vi "Main.vi"() -> ()   [LabVIEW 2016]
uses:
  <vilib>/Platform/TimedLoop/XDataNode/timing_clust.ctl
  <vilib>/Platform/TimedLoop/XDataNode/nitl_modes.ctl
  <vilib>/Platform/TimedLoop/XDataNode/wakeup.ctl
  <vilib>/rvi/Emulation/niFpgaGetClockAttributes.vi
  <vilib>/rvi/Emulation/niFpgaSctlEmulationGetInTimedLoop.vi
  <vilib>/rvi/Emulation/niFpgaEmulationReportErrorSimple.vi
  <vilib>/rvi/Emulation/niFpgaCriticalErrorInLSC.vi
  <vilib>/rvi/Emulation/niFpgaEmulationIsFPGAContextNoSignature.vi
  <vilib>/rvi/DataTransferAndStorage/Container/Common/niFpgaContainerGetUniqueNameForEmu.vi
  <vilib>/rvi/Memory/Memory_Emulation/niFpgaMemoryEmulationCacheClearOnFirstRun.vi
  <vilib>/rvi/Memory/Memory_Emulation/nirvimemoryEmulationManagerCache_MakeExclusive.vi
  <vilib>/rvi/Memory/Memory_Emulation/niFpgaMemoryEmulationValidateCache.vi
  <vilib>/rvi/Memory/Memory_Emulation/nirvimemoryEmulationManagerCache_InsertValue.vi
  <vilib>/Utility/error.llb/Clear Errors.vi
  <vilib>/rvi/Memory/Memory_Emulation/nirvimemoryEmulationManagerCache_ReleaseExclusive.vi
  <vilib>/rvi/Memory/Memory_Emulation/nirvimemoryEmulationManagerCache_GetValue.vi
  <vilib>/rvi/Memory/Memory_Emulation/nirvimemoryEmulationManagerCache_SetValue.vi
  <vilib>/rvi/Emulation/niFpgaProcessEmulError.vi
  <vilib>/rvi/Memory/Memory_Emulation/nirvimemoryFastEmulation.vi
  <vilib>/rvi/Memory/Memory_Emulation/nirvimemoryEmulation.vi
  <vilib>/rvi/errors/nirviReportUnexpectedCaseInternalError (U32).vi
  <vilib>/rvi/DataTransferAndStorage/Container/Common/niFpgaContainerExecOnDevCompGetState.vi
  <vilib>/rvi/Emulation/niFpgaSctlEmulationResourceMgr.vi
  <vilib>/Platform/TimedLoop/XDataNode/XDataNode.xnode
  <vilib>/rvi/DataTransferAndStorage/Container/XNode/niFpgaContainer.xnode
  <vilib>/rvi/DataTransferAndStorage/Register/Emulation/niFpgaRegisterEmulation.vi
  <vilib>/rvi/Memory/Memory_Emulation/niFpgaMemoryEmulationRefIn.vi
  <vilib>/Platform/TimedLoop/XDataNode/XDNodeRunTimeDep.lvlib
panel:
  out "Flags":u8
  out "InclinometerAngle":u32
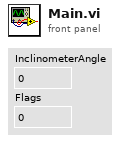
[diagram p1: front panel]
types:
  T1 = typedef "XDNodeRunTimeDep.lvlib/timing_clust.ctl" = cluster{"Expected End [f-1]":u64, "Actual End [f-1]":u64, "Finished Late? [f-1]":bool, "Expected End [i-1]":u64, "Actual End [i-1]":u64, "Finished Late? [i-1]":bool, "Expected Start [i]":u64, "Actual Start [i]":u64, "Expected Start [f]":u64, "Actual Start [f]":u64, "Source Name":string, "Structure Name":string, "Period":i64, "Deadline":i64, "Offset":i64, "Start":i64, "Priority":i32, "Timeout":i32, "Mode":T2, "Wakeup Reason":T3, "Error":errorcluster, "Source Type":string, "Secondary Source Type":string, "Global End Time":u64, "Global Start Time":u64, "Frame Duration":u64, "Iteration Duration":u64, "Assigned CPU":i32, "I/O Scan Engine Mode":u32}
  T2 = typedef "XDNodeRunTimeDep.lvlib/nitl_modes.ctl" = enum32{"No Change", "Process missed periods, maintain original phase", "Discard missed periods, maintain original phase", "Process missed periods, ignore original phase", "Discard missed periods, ignore original phase"}
  T3 = typedef "XDNodeRunTimeDep.lvlib/wakeup.ctl" = enum32{"Normal", "Aborted", "Asynchronous wakeup", "Timing source error", "Timed loop error", "Timeout"}
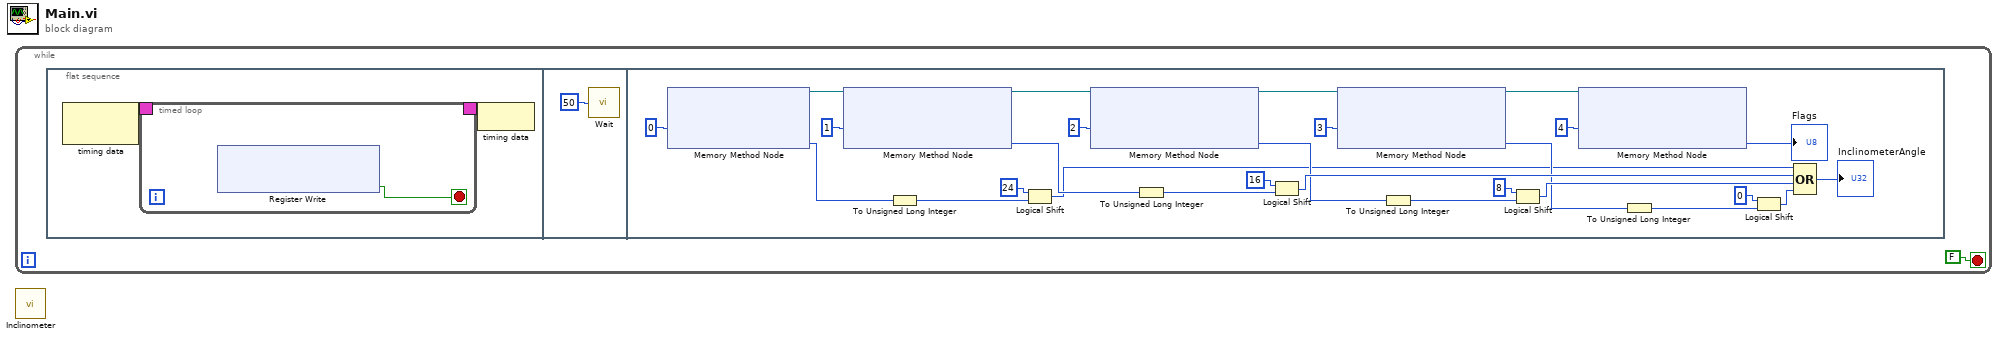
[diagram p0: block diagram]
diagram:
  n1 = while {
    stop <- FALSE stop-if-true
    n2 = flat-sequence {
      frame #0 {
        n3 = node-c288() -> (w3:T1)  [unwired: 1 in]
        n4 = timed-loop {
          timing: w3 -> [_]
          timing-out: [_] -> w2
          stop <- w4 stop-if-true
          n5 = xnode "Register Write"() -> ("Data"=w4:bool)  [unwired: 1 in, 1 out]
        }
        n6 = node-c288(w2) -> ()
      }
      frame #1 {
        n7 = call "Wait"("Count(mSec)"=u32 50) -> ()  [unwired: 1 out]
      }
      frame #2 {
        n8 = xnode ("Memory Method Node")("Address"=u32 0) -> ("Data"=w21:u8, "Memory Out"=w18:refnum<k21>)  [unwired: 1 in]
        n9 = xnode ("Memory Method Node")("Address"=u32 1, "Memory In"=w18) -> ("Data"=w22:u8, "Memory Out"=w19:refnum<k21>)
        n10 = To Unsigned Long Integer(number=w21) -> (unsigned 32bit integer=w13:u32)
        n11 = Logical Shift(y=i16 24, x=w13) -> (x << y=w11:u32)
        n12 = xnode ("Memory Method Node")("Address"=u32 2, "Memory In"=w19) -> ("Data"=w24:u8, "Memory Out"=w20:refnum<k21>)
        n13 = To Unsigned Long Integer(number=w22) -> (unsigned 32bit integer=w23:u32)
        n14 = Logical Shift(y=i16 16, x=w23) -> (x << y=w30:u32)
        n15 = xnode ("Memory Method Node")("Address"=u32 3, "Memory In"=w20) -> ("Data"=w26:u8, "Memory Out"=w34:refnum<k21>)
        n16 = To Unsigned Long Integer(number=w24) -> (unsigned 32bit integer=w25:u32)
        n17 = Logical Shift(y=i16 8, x=w25) -> (x << y=w32:u32)
        n18 = xnode ("Memory Method Node")("Address"=u32 4, "Memory In"=w34) -> ("Data"=→"Flags":u8)  [unwired: 1 out]
        n19 = To Unsigned Long Integer(number=w26) -> (unsigned 32bit integer=w27:u32)
        n20 = Logical Shift(y=i16 0, x=w27) -> (x << y=w31:u32)
        n21 = Compound Arithmetic op=OR(w11, w30, w32, w31) -> (→"InclinometerAngle":u32)
      }
    }
  }
  n22 = call "Inclinometer.vi"() -> ()  [unwired: 12 in]
